vi "LED flash.vi"() -> ()   [LabVIEW 2011]
uses:
  <vilib>/rvi/eio/common/nirviEmuTemplateMethod_errors.vi
  <vilib>/eio/EIONode/EIONode.xnode
panel:
  out "Chassis Temperature":i16
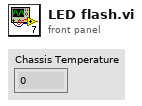
[diagram p1: front panel]
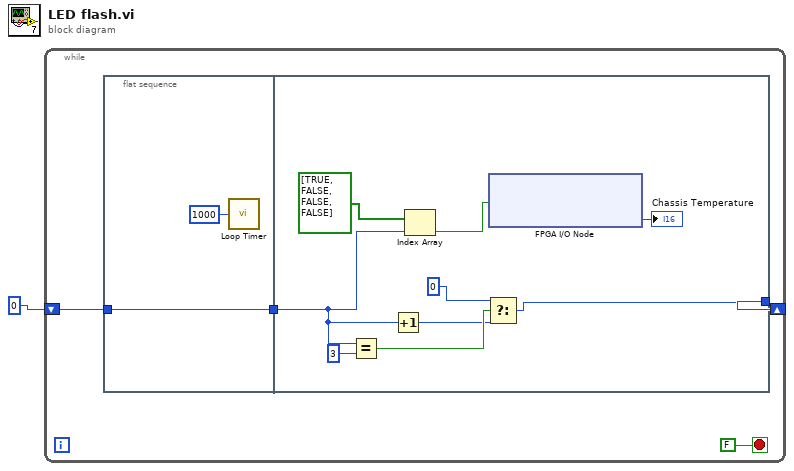
[diagram p0: block diagram]
diagram:
  n1 = while {
    shift-right: [w3] -> _
    shift-left: i16 0 -> [w4]
    stop <- FALSE stop-if-true
    n2 = flat-sequence {
      tunnel: [w6] -> w5
      tunnel: w4 -> [w6]
      tunnel: w5 -> [w14]
      tunnel: [w12] -> w3
      frame #0 {
        n3 = call "Loop Timer"("Count(mSec)"=u32 1000) -> ()  [unwired: 1 out]
      }
      frame #1 {
        n4 = Equal?(x=w14, y=i16 3) -> (x = y?=w11:bool)
        n5 = Increment(x=w14) -> (x+1=w9:i16)
        n6 = Index Array(array=bool[] [TRUE, FALSE, FALSE, FALSE], index=w14) -> (element=w15:bool)
        n7 = Select(t=i16 0 ("y"), s=w11, f=w9) -> (s? t:f=w12:i16)
        n8 = xnode "FPGA I/O Node"("FPGA LED"=w15) -> ("Chassis Temperature"=→"Chassis Temperature":i16)  [unwired: 2 in, 2 out]
      }
    }
  }
